vi "WT500 Read Power.vi"(0 "VISA resource name":refnum<visa-resource-name>="WT500", 1 "WT500 CMDS":T1, 5 "V Range (8: 1000V)":u16(ring)=6 items=["AUTO", "15", "30", "60", "100", "150", "300", "600", "1000", "7.5", "15", "30", "50", "75", "150", "300", "500"], 7 "I Range (7: 40A)":u16(ring)=7 items=["AUTO", "500 mA", "1 A", "2 A", "5 A", "10 A", "20 A", "40 A", "S-AUTO", "50 mV", "100 mV", "200 mV", "500 mV", "1 V", "2 V", "5 V", "10 V", "250 mA", "500 mA", "1 A", "2.5 A", "5 A", "10 A", "20 A", "25 mV", "50 mV", "100 mV", "250 mV", "500 mV", "1 V", "2.5 V", "5 V"], 11 "error in (no error)":errorcluster) -> (4 "VISA resource name out":refnum<visa-resource-name>="WT500", 6 "PowerData":T2={"Current L1"=236.2, "Current L2"=17.749, "Power"=4192.0, "WattHours"=0.0}, 8 "Error Message":string, 10 "Measurement Values":dbl[](array[numeric]) format="%.4p", 14 "Label":string[](array[string])=["Urms:Element 1", "Urms:Element 2", "Irms:Element 1", "Irms:Element 2", "P:Sigma", "Wp:Sigma", "I +peak:Element 1", "I +peak:Element 2"], 15 "error out":errorcluster)   [LabVIEW 2016]
uses:
  Drivers/Yokogawa WT500/Type Definitions/WT500 Dryer Power Data.ctl
  Drivers/Yokogawa WT500/Type Definitions/WT500 Sequences.ctl
  Drivers/Yokogawa WT500/LLBs/ykwt500.llb/YKWT500 Configure Numeric Item (Set).vi
panel:
  out "(Max Current)":dbl
  in  "Pole":u16(ring)=1 items=["NONE", "Element 1", "Element 2", "Element 3", "Sigma"]
  in  "Measurement":u16(ring)=1 items=["None", "Urms", "Umn", "Udc", "Urmn", "Uac", "Irms", "Imn", "Idc", "Irmn", "Iac", "P", "S", "Q", "Lambda", "Phi", "Freq U", "Freq I", "U +peak", "U -peak", "I +peak", "I -peak", "Cf U", "Cf I", "Time", "Wp", "Wp+", "Wp-", "q", "q+", "q-", "WS", "WQ", "Eta 1", "Eta 2", "F1", "F2", "F3", "F4", "F5", "F6", "F7", "F8", "U(k)", "I(k)", "P(k)", "S(k)", "Q(k)", "Lambda(k)", "Phi(k)", "Phi U(k)", "Phi I(k)", "Uhdf(k)", "Ihdf(k)", "Phdf(k)", "Uthd", "Ithd", "Pthd", "Phi Ui-Uj", "Phi Ui-Uk", "Phi Ui-Ii", "Phi Ui-Ij", "Phi Ui-Ik", "Delta 1", "Delta 2", "Delta 3", "Delta 4"]
  out "Data Length":i32
  out "Read Data":string
  in  "Write Data":string
  out "Scan Error":bool
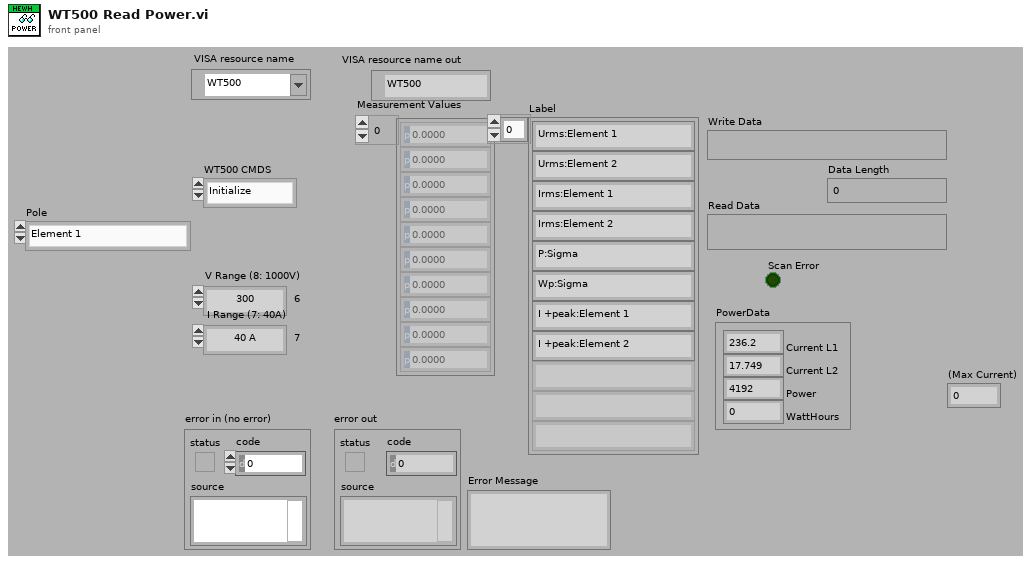
[diagram p1: front panel]
types:
  T1 = typedef "WT500 Sequences.ctl" = enum16{"Initialize", "GetReadings", "GetErrors", "Close", "NoOp", "MiscCmd"}
  T2 = typedef "WT500 Dryer Power Data.ctl" = cluster{"Current L1":dbl, "Current L2":dbl, "Power":dbl, "WattHours":dbl}
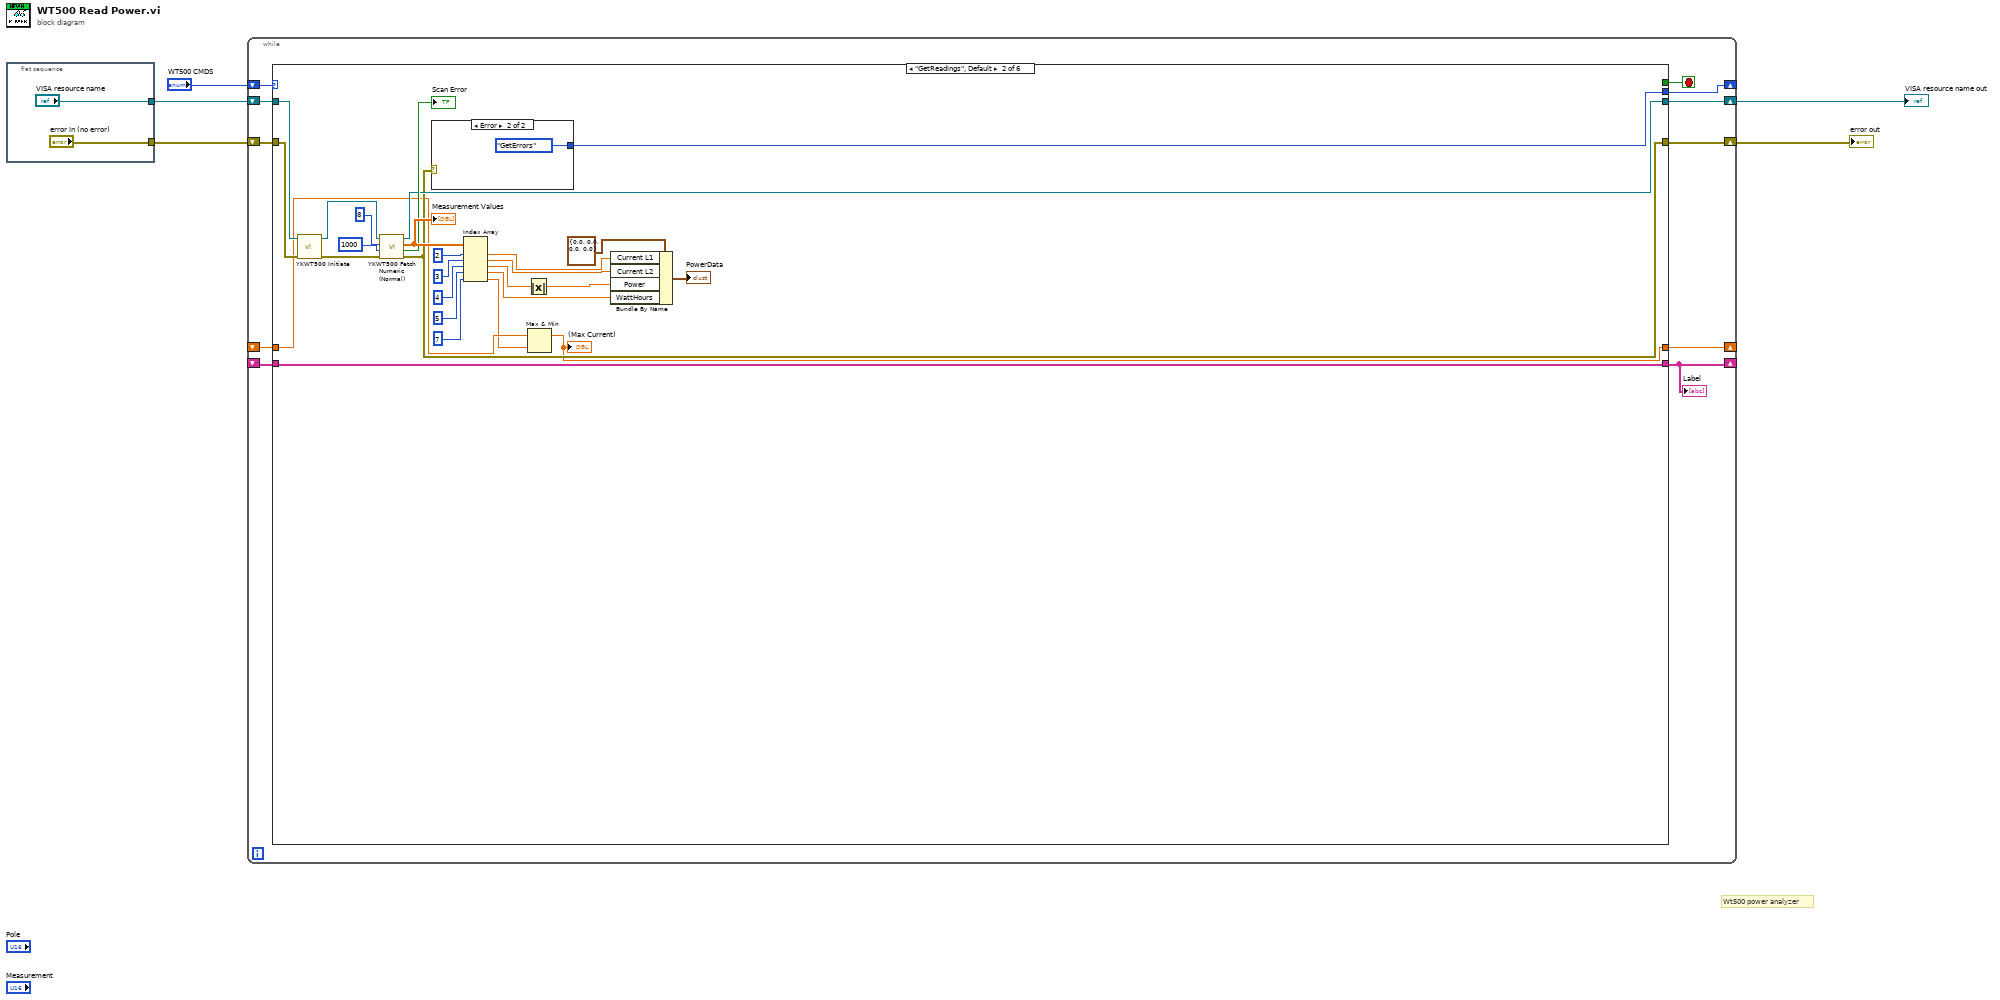
[diagram p0: block diagram]
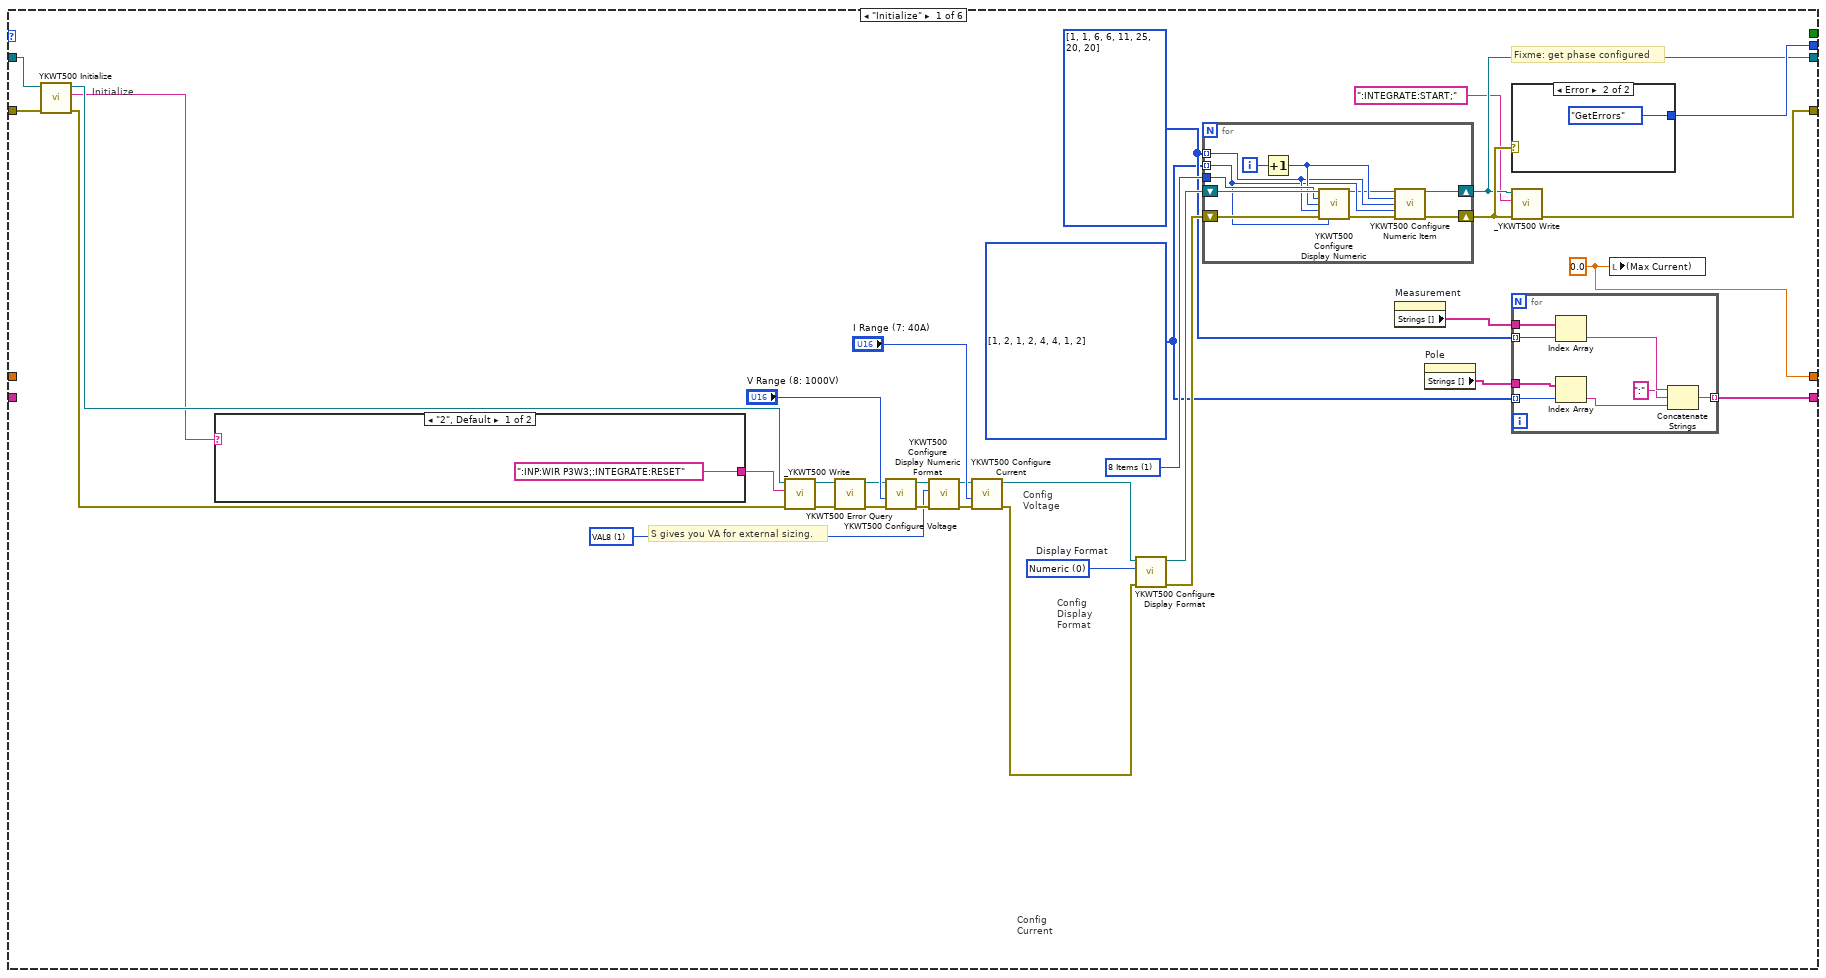
[diagram p2: hidden frame]
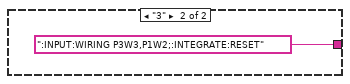
[diagram p3: hidden frame]
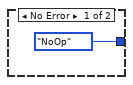
[diagram p4: hidden frame]
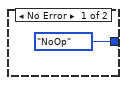
[diagram p5: hidden frame]
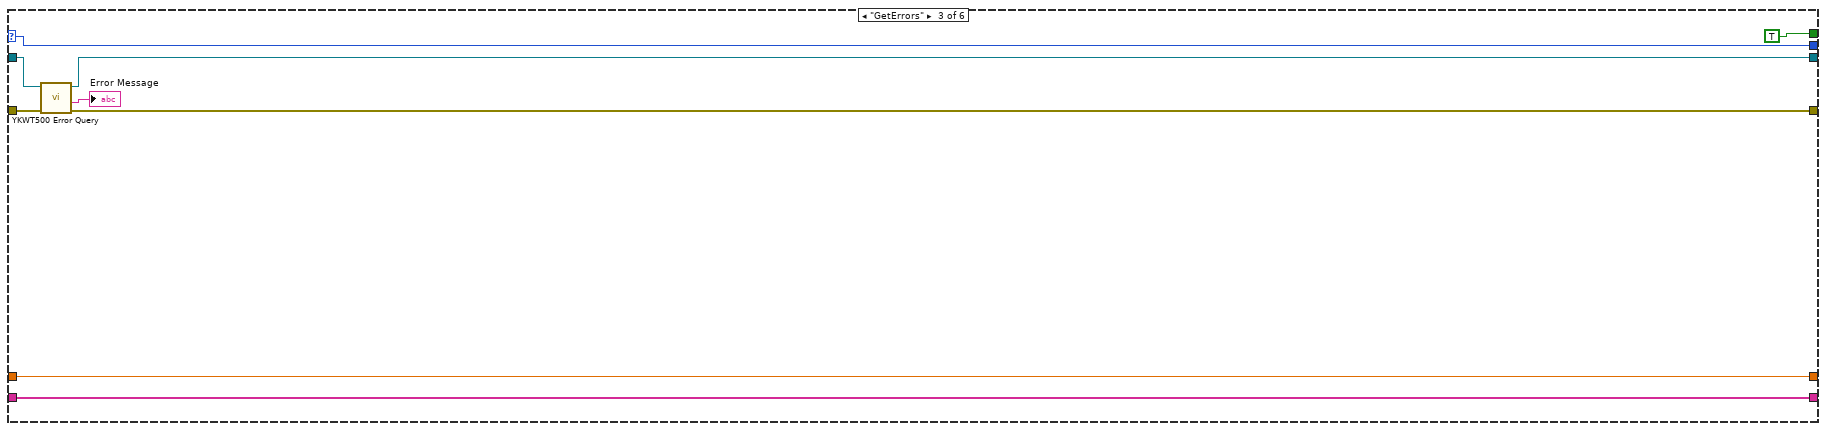
[diagram p6: hidden frame]
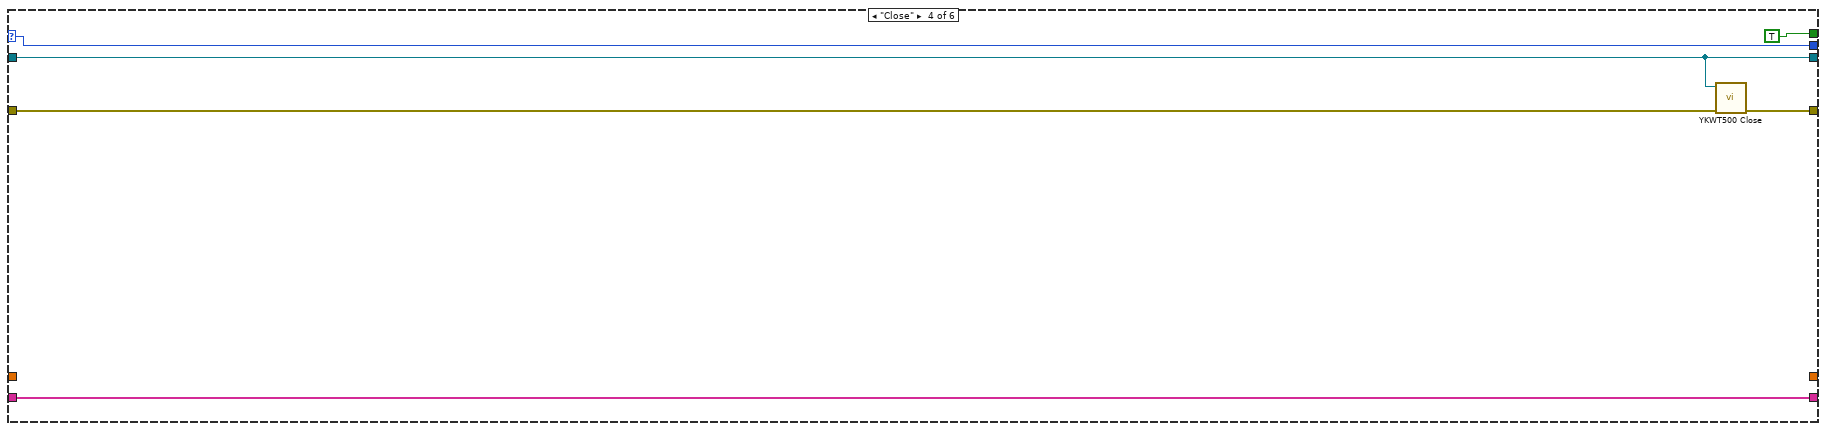
[diagram p7: hidden frame]
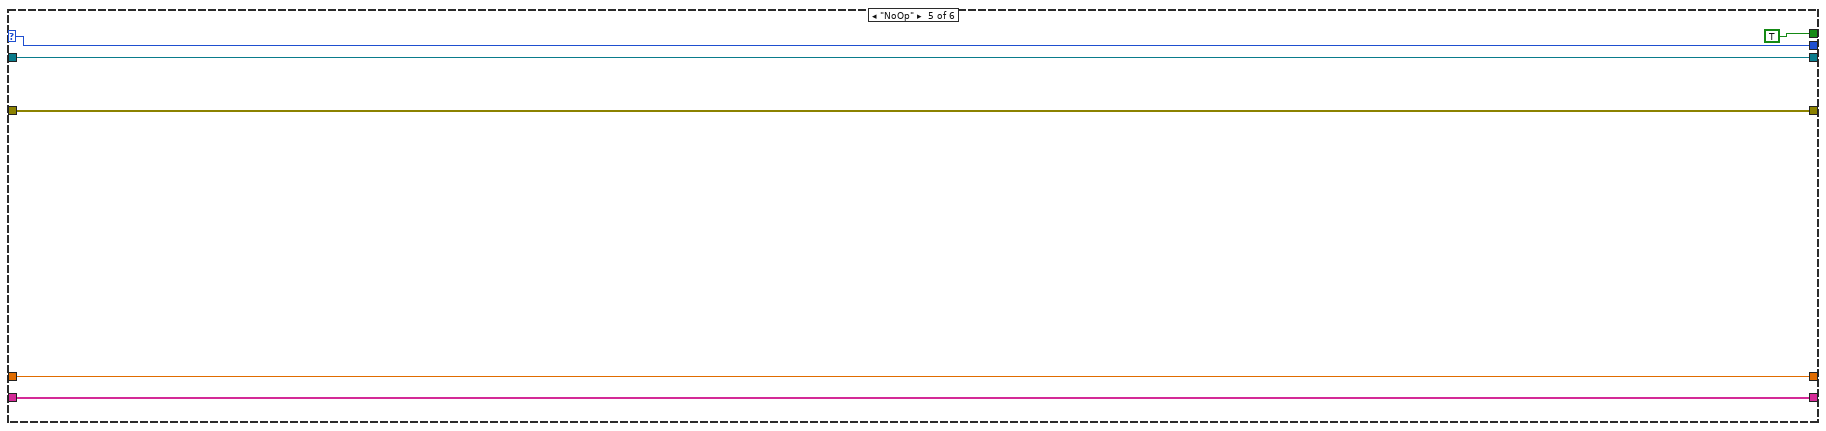
[diagram p8: hidden frame]
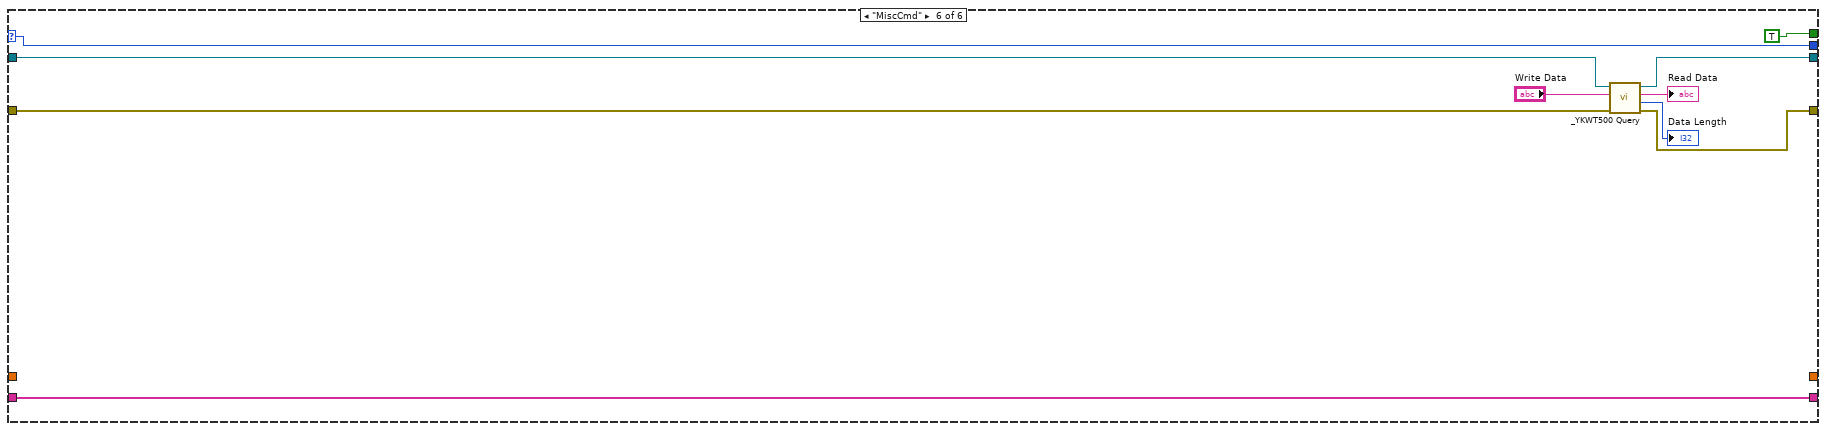
[diagram p9: hidden frame]
diagram:
  # "Wt500 power analyzer"
  n1 = flat-sequence {
    tunnel: ["error in (no error)"] -> w2
    tunnel: ["VISA resource name"] -> w1
    frame #0 {
    }
  }
  n2 = while {
    shift-right: [w16] -> w4
    shift-left: w2 -> [w17]
    shift-right: [w14] -> _
    shift-left: "WT500 CMDS" -> [w18]
    shift-right: [w12] -> w3
    shift-left: w1 -> [w13]
    shift-right: [w10] -> _
    shift-left: _ -> [w11]
    shift-right: [w9] -> _
    shift-left: _ -> [w8]
    stop <- w15 stop-if-true
    n3 = case shown="\"GetReadings\", Default" w18 {
      selector: w18 -> [_ _ w109 w116 w123 w134]
      tunnel: w17 -> [w47 w83 w111 w119 w124 w131]
      tunnel: [w27 w86 w107 w118 w124 w130] -> w16
      tunnel: [_ _ TRUE TRUE TRUE TRUE] -> w15
      tunnel: [w46 w85 w109 w116 w123 w134] -> w14
      tunnel: w13 -> [w45 w84 w113 w117 w122 w133]
      tunnel: [w28 w87 w112 w117 w122 w132] -> w12
      tunnel: [w34 w80 w106 w114 w121 w126] -> w10
      tunnel: w11 -> [_ w80 w106 w114 w121 w126]
      tunnel: [w30 w76 w105 _ w120 _] -> w9
      tunnel: w8 -> [_ w78 w105 _ w120 _]
      frame "Initialize" {
        w19 = u16[] [1, 2, 1, 2, 4, 4, 1, 2] items=["NONE", "Element 1", "Element 2", "Element 3", "Sigma"]
        w20 = u16[] [1, 1, 6, 6, 11, 25, 20, 20] items=["None", "Urms", "Umn", "Udc", "Urmn", "Uac", "Irms", "Imn", "Idc", "Irmn", "Iac", "P", "S", "Q", "Lambda", "Phi", "Freq U", "Freq I", "U +peak", "U -peak", "I +peak", "I -peak", "Cf U", "Cf I", "Time", "Wp", "Wp+", "Wp-", "q", "q+", "q-", "WS", "WQ", "Eta 1", "Eta 2", "F1", "F2", "F3", "F4", "F5", "F6", "F7", "F8", "U(k)", "I(k)", "P(k)", "S(k)", "Q(k)", "Lambda(k)", "Phi(k)", "Phi U(k)", "Phi I(k)", "Uhdf(k)", "Ihdf(k)", "Phdf(k)", "Uthd", "Ithd", "Pthd", "Phi Ui-Uj", "Phi Ui-Uk", "Phi Ui-Ii", "Phi Ui-Ij", "Phi Ui-Ik", "Delta 1", "Delta 2", "Delta 3", "Delta 4"] ("Array of Measurements")
        w30 = 0.0
        w37 = u16 1 items=["VAL4", "VAL8", "VAL16", "MATRIX", "ALL"] ("Display Format (0: Numeric)")
        w42 = u16 1 items=["4 Items", "8 Items", "16 Items", "Matrix"] ("Numeric Format (0: 4 Items)")
        w52 = u16 0 items=["Numeric", "Wave", "Bar", "Vector", "Trend"]  # Display Format
        # "S gives you VA for external sizing."
        # "Fixme: get phase configured"
        # "Config\nDisplay\nFormat"
        # "Config\nCurrent"
        # "Config\nVoltage"
        # "Initialize"
        n4 = call "YKWT500 Initialize.vi"("error in (no error)"=w47, "VISA resource name"=w45) -> ("error out"=w32:errorcluster, "Instrument ID"=w21:string, "VISA resource name out"=w33:refnum<visa-resource-name>)  [unwired: 7 in]
        n5 = case shown="\"2\", Default" w21 {
          tunnel: [":INP:WIR P3W3;:INTEGRATE:RESET" ("Write Data") ":INPUT:WIRING P3W3,P1W2;:INTEGRATE:RESET" ("Write Data")] -> w31
          frame "2", Default {
          }
          frame "3" {
          }
        }
        n6 = call "_YKWT500 Write.vi"("error in (no error)"=w32, "Write Data"=w31, "VISA resource name"=w33) -> ("error out"=w25:errorcluster, "VISA resource name out"=w24:refnum<visa-resource-name>)  [unwired: 5 in, 2 out]
        n7 = call "YKWT500 Error Query.vi"("error in (no error)"=w25, "VISA resource name"=w24) -> ("error out"=w22:errorcluster, "VISA resource name out"=w23:refnum<visa-resource-name>)  [unwired: 6 in, 2 out]
        n8 = call "YKWT500 Configure Voltage.vi"("error in (no error)"=w22, "Voltage Range (8: 1000V)"="V Range (8: 1000V)", "VISA resource name"=w23) -> ("error out"=w41:errorcluster, "VISA resource name out"=w38:refnum<visa-resource-name>)  [unwired: 7 in]
        n9 = call "YKWT500 Configure Display Numeric Format.vi"("error in (no error)"=w41, "Numeric Format (0: 4 Items)"=w37, "VISA resource name"=w38) -> ("error out"=w40:errorcluster, "VISA resource name out"=w39:refnum<visa-resource-name>)  [unwired: 7 in]
        n10 = call "YKWT500 Configure Current.vi"("error in (no error)"=w40, "Current Range (7: 40A)"="I Range (7: 40A)", "VISA resource name"=w39) -> ("error out"=w51:errorcluster, "VISA resource name out"=w50:refnum<visa-resource-name>)  [unwired: 7 in]
        n11 = call "YKWT500 Configure Display Format.vi"("error in (no error)"=w51, "Display Format (0: Numeric)"=w52, "VISA resource name"=w50) -> ("error out"=w43:errorcluster, "VISA resource name out"=w44:refnum<visa-resource-name>)  [unwired: 7 in]
        n12 = for {
          shift-right: [w65] -> w28
          shift-left: w44 -> [w73]
          shift-right: [w63] -> w29
          shift-left: w43 -> [w72]
          tunnel: w42 -> [w70]
          tunnel: w19 -> [w67] mode=indexing
          tunnel: w20 -> [w68] mode=indexing
          i -> [w71]
          n13 = Increment(x=w71) -> (x+1=w69:i32)
          n14 = call "YKWT500 Configure Display Numeric.vi"("VISA resource name"=w73, "Numeric Format (0: 4 Items)"=w70, "Numeric Item Number (1)"=w69, "Numeric Function (0: None)"=w68, "error in (no error)"=w72, "Element (1: Element 1)"=w67) -> ("VISA resource name out"=w66:refnum<visa-resource-name>, "error out"=w64:errorcluster)  [unwired: 8 in]
          n15 = call-poly "YKWT500 Configure Numeric Item.vi"("VISA resource name"=w66, "Numeric Item Number (1)"=w69, "Numeric Function (0: None)"=w68, "Element (1: Element 1)"=w67, "error in (no error)"=w64) -> ("VISA resource name out"=w65:refnum<visa-resource-name>, "error out"=w63:errorcluster)  [unwired: 9 in]
        }
        n16 = property on="Measurement" class="Ring (strict)"() -> ("Strings []"=w36:string[])  [unwired: 2 in, 2 out]
        n17 = property on="Pole" class="Ring (strict)"() -> ("Strings []"=w35:string[])  [unwired: 2 in, 2 out]
        n18 = case shown="Error" w29 {
          tunnel: [WT500_Sequences."NoOp" ("WT500 CMDS") WT500_Sequences."GetErrors" ("WT500 CMDS")] -> w46
          frame No Error {
          }
          frame Error {
          }
        }
        n19 = call "_YKWT500 Write.vi"("error in (no error)"=w29, "Write Data"=":INTEGRATE:START;", "VISA resource name"=w28) -> ("error out"=w27:errorcluster)  [unwired: 5 in, 3 out]
        n20 = for {
          tunnel: w20 -> [w62] mode=indexing
          tunnel: w36 -> [w61]
          tunnel: w19 -> [w60] mode=indexing
          tunnel: w35 -> [w59]
          tunnel: [w55] -> w34 mode=indexing
          n21 = Index Array(array=w61, index=w62) -> (element=w58:string)
          n22 = Index Array(array=w59, index=w60) -> (element=w56:string)
          n23 = Concatenate Strings(w58, ":" ("string"), w56) -> (w55:string)
        }
        n24 = local write "(Max Current)"(w30) -> ()
      }
      frame "GetReadings", Default {
        n25 = call "YKWT500 Initiate.vi"("error in (no error)"=w83, "VISA resource name"=w84) -> ("error out"=w81:errorcluster, "VISA resource name out"=w82:refnum<visa-resource-name>)  [unwired: 8 in]
        n26 = call "YKWT500 Fetch Numeric (Normal).vi"("error in (no error)"=w81, "Timeout (10000 ms)"=u32 1000, "Number of Item (255)"=8, "VISA resource name"=w82) -> ("error out"=w86:errorcluster, "Scan Error"=→"Scan Error":bool, "Measurement Value"=w91:dbl[], "VISA resource name out"=w87:refnum<visa-resource-name>)  [unwired: 4 in]
        "Measurement Values" <- w91
        n27 = case shown="Error" w86 {
          tunnel: [WT500_Sequences."NoOp" ("WT500 CMDS") WT500_Sequences."GetErrors" ("WT500 CMDS")] -> w85
          frame No Error {
          }
          frame Error {
          }
        }
        n28 = Index Array(array=w91, index #1=2 ("index"), index #2=3 ("index"), index #3=4 ("index"), index #4=5 ("index"), index #5=7 ("index")) -> (element #1=w101:dbl, element #2=w100:dbl, element #3=w95:dbl, element #4=w98:dbl, element #5=w77:dbl)
        n29 = Absolute Value(x=w95) -> (abs(x)=w99:dbl)
        n30 = Max & Min(x=w78, y=w77) -> (max(x,y)=w76:dbl)  [unwired: 1 out]
        "(Max Current)" <- w76
        n31 = Bundle By Name(cluster=T2 {"Current L1"=0.0, "Current L2"=0.0, "Power"=0.0, "WattHours"=0.0} ("PowerData"), "Current L1"=w101, "Current L2"=w100, "Power"=w99, "WattHours"=w98) -> (→"PowerData":T2)
      }
      frame "GetErrors" {
        n32 = call "YKWT500 Error Query.vi"("error in (no error)"=w111, "VISA resource name"=w113) -> ("error out"=w107:errorcluster, "Error Message"=→"Error Message":string, "VISA resource name out"=w112:refnum<visa-resource-name>)  [unwired: 6 in, 1 out]
      }
      frame "Close" {
        n33 = call "YKWT500 Close.vi"("error in (no error)"=w119, "VISA resource name"=w117) -> ("error out"=w118:errorcluster)  [unwired: 9 in]
      }
      frame "NoOp" {
      }
      frame "MiscCmd" {
        n34 = call "_YKWT500 Query.vi"("error in (no error)"=w131, "Write Data"="Write Data", "VISA resource name"=w133) -> ("error out"=w130:errorcluster, "Data Length"=→"Data Length":i32, "Read Data"=→"Read Data":string, "VISA resource name out"=w132:refnum<visa-resource-name>)  [unwired: 5 in]
      }
    }
    "Label" <- w10
  }
  "error out" <- w4
  "VISA resource name out" <- w3
